vi "TestObserveU32_ValueOne.vi"(8 "error in (no error)":errorcluster, 11 "TestCase in":refnum<class "TestObservableData.lvclass">) -> (0 "error out":errorcluster, 3 "TestCase out":refnum<class "TestObservableData.lvclass">)   [LabVIEW 2015, in "TestObservableData.lvclass"]
uses:
  TestObservableData.lvclass
  TestObservableData.lvclass/TestObservableData.ctl
  Framework/SubscriptionPolicy/BasicSubscription/BasicSubscription.lvclass/BasicSubscription.ctl
  Framework/IMediator/SubscriptionRequest/SubscriptionRequest.lvclass/SubscriptionRequest.ctl
  Framework/IMediator/IMediator Messages/Subscribe Msg/Subscribe Msg.lvclass/Subscribe Msg.ctl
  <vilib>/ActorFramework/Message Enqueuer/Message Enqueuer.lvclass/Message Enqueuer.ctl
  <vilib>/ActorFramework/Message Enqueuer/Enqueue.vi
  <vilib>/ActorFramework/Message Priority Queue/Priority Enqueue.vi
  Framework/SubscriptionPolicy/BasicSubscription/BasicSubscription.lvclass
  Framework/IMediator/SubscriptionRequest/SubscriptionRequest.lvclass
  Framework/IMediator/IMediator Messages/Subscribe Msg/Subscribe Msg.lvclass
  Framework/IMediator/ISubscriptionPolicy/ISubscriptionPolicy.lvclass
  Framework/Transport/TerminalBinding/TerminalBinding.lvclass
panel:
  out "ControlTerminal":u32
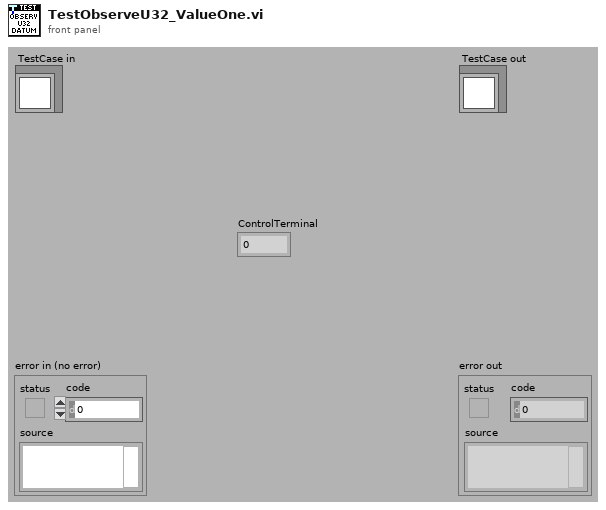
[diagram p1: front panel]
types:
  T1 = typedef "IMediator.lvlib/ISubscriptionPolicy.lvclass/ISubscriptionPolicy Reference.ctl" = refnum<data-value>
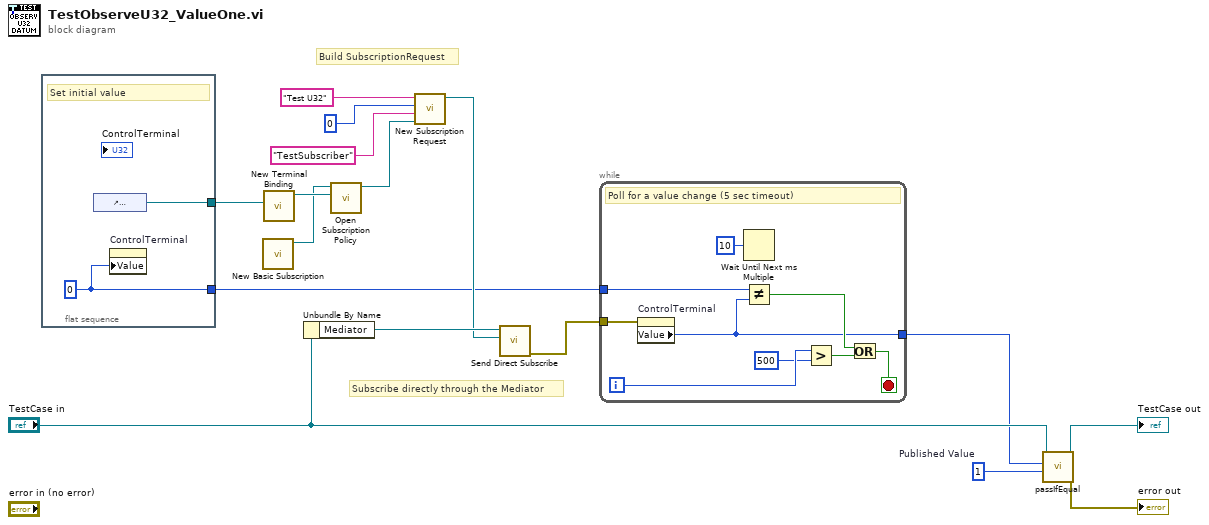
[diagram p0: block diagram]
diagram:
  w2 = u32 1  # Published Value
  # "Build SubscriptionRequest"
  # "Subscribe directly through the Mediator"
  n1 = flat-sequence {
    tunnel: [w18] -> w6
    tunnel: [w17] -> w4
    frame #0 {
      w17 = u32 0 ("ControlTerminal")
      # "Set initial value"
      n2 = control-ref of="ControlTerminal"() -> (w18:refnum<vi>)
      n3 = property on="ControlTerminal" class="DigNum (strict)"("Value"=w17) -> ()  [unwired: 2 in, 2 out]
    }
  }
  n4 = call "New Basic Subscription.vi"() -> ("BasicSubscription Out"=w1:refnum<class "BasicSubscription.lvclass">)  [unwired: 11 in]
  n5 = call "New Terminal Binding.vi"("Ctl Refnum"=w6) -> ("TerminalBinding"=w7:refnum<class "TerminalBinding.lvclass">)  [unwired: 9 in, 1 out]
  n6 = Unbundle By Name("TestCase in") -> ("Mediator"=w13:refnum<class "Message Enqueuer.lvclass">)
  n7 = call "Open Subscription Policy.vi"("Transport"=w7, "SubscriptionPolicy"=w1) -> ("Subscription Policy"=w8:T1)  [unwired: 8 in, 1 out]
  n8 = call "New Subscription Request.vi"("Subscription Policy"=w8, "Subscriber ID"="TestSubscriber" ("Unique Subscriber ID"), "Type"=u32 0, "Datum Name"="Test U32" ("Topic Name")) -> ("SubscriptionRequest"=w12:refnum<class "SubscriptionRequest.lvclass">)  [unwired: 7 in]
  n9 = call "Send Direct Subscribe.vi"("Subscription Request"=w12, "Message Enqueuer"=w13) -> ("error out"=w5:errorcluster)  [unwired: 8 in, 1 out]
  n10 = while {
    tunnel: w5 -> [w27]
    tunnel: w4 -> [w26]
    tunnel: [w19] -> w3
    i -> [w22]
    stop <- w20 stop-if-true
    # "Poll for a value change (5 sec timeout)"
    n11 = property on="ControlTerminal" class="DigNum (strict)"(error in=w27) -> ("Value"=w19:u32)  [unwired: 1 in, 2 out]
    n12 = Wait Until Next ms Multiple(millisecond multiple=u32 10 ("milliseconds to wait")) -> ()  [unwired: 1 out]
    n13 = Not Equal?(x=w26, y=w19) -> (x != y?=w25:bool)
    n14 = Greater?(x=w22, y=500) -> (0:w23:bool)
    n15 = Or(x=w25, y=w23) -> (x .or. y?=w20:bool)
  }
  n16 = call-dynamic "passIfEqual.vi"("y"=w2, "x"=w3, "TestCase in"="TestCase in") -> ("error out"=→"error out":errorcluster, "TestCase out"=→"TestCase out":refnum<class "TestObservableData.lvclass">)  [unwired: 7 in]
